vi "Convert T to R.vi"(10 "SH Coeff":cluster{"A":dbl, "B":dbl, "C":dbl}={"A"=0.0010291947674, "B"=0.0002391275184, "C"=1.5662771497e-07}, 11 "T":dbl=25.0 caption="T (degC)") -> (3 "R":dbl=10000.000000163434 caption="R (Ohms)")   [LabVIEW 2014, in "Temperature.lvlib"]
doc: "Convert a temperature in degrees Celsius to a thermister resistance in Ohms for a particular thermistor model given the Steinhart-Hart coefficients for that thermistor."
uses:
  Temperature.lvlib
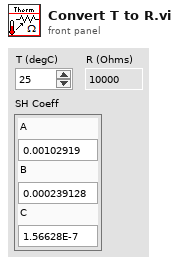
[diagram p1: front panel]
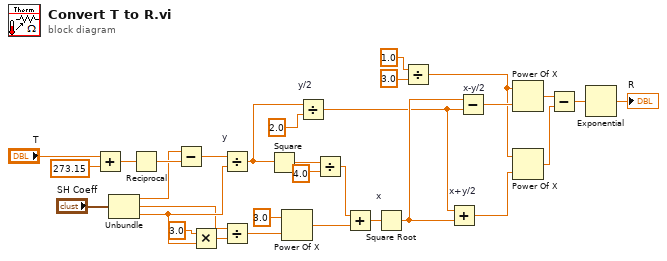
[diagram p0: block diagram]
diagram:
  n1 = Add(x="T", y=273.15) -> (x+y=w29:dbl)
  n2 = Unbundle("SH Coeff") -> ("A"=w3:dbl, "B"=w1:dbl, "C"=w2:dbl)
  n3 = Reciprocal(x=w29) -> (1/x=w28:dbl)
  n4 = Subtract(x=w3, y=w28) -> (x-y=w27:dbl)
  n5 = Multiply(x=3.0, y=w2) -> (x*y=w25:dbl)
  n6 = Divide "y"(x=w27, y=w2) -> (x/y=w17:dbl)
  n7 = Divide ("y")(x=w1, y=w25) -> (x/y=w23:dbl)
  n8 = Square(x=w17) -> (x^2=w22:dbl)
  n9 = Power Of X(1:w23, 2:3.0 ("y")) -> (0:w19:dbl)
  n10 = Divide "y/2"(x=w17, y=2.0) -> (x/y=w5:dbl)
  n11 = Divide ("y")(x=w22, y=4.0) -> (x/y=w20:dbl)
  n12 = Add(x=w20, y=w19) -> (x+y=w18:dbl)
  n13 = Square Root "x"(x=w18) -> (sqrt(x)=w6:dbl)
  n14 = Divide(x=1.0, y=3.0) -> (x/y=w11:dbl)
  n15 = Add "x+y/2"(x=w5, y=w6) -> (x+y=w15:dbl)
  n16 = Subtract "x-y/2"(x=w6, y=w5) -> (x-y=w12:dbl)
  n17 = Power Of X(1:w12, 2:w11) -> (0:w10:dbl)
  n18 = Power Of X(1:w15, 2:w11) -> (0:w9:dbl)
  n19 = Subtract(x=w10, y=w9) -> (x-y=w8:dbl)
  n20 = Exponential(1:w8) -> (0:→"R":dbl)
